vi "Test MQTT-7.1.2-1.vi"(8 "error in (no error)":errorcluster) -> (0 "error out":errorcluster)   [LabVIEW 2013]
uses:
  <vilib>/addons/_JKI Toolkits/Caraya/classes/Test/Test.lvclass
  source/Client/Client.lvclass
  source/MQTT_Base/MQTT_Base.lvclass
  <vilib>/addons/_JKI Toolkits/Caraya/classes/Assert/Assert.lvclass
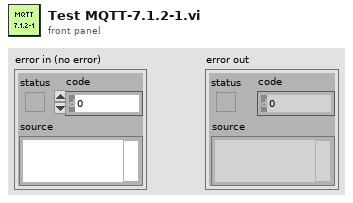
[diagram p1: front panel]
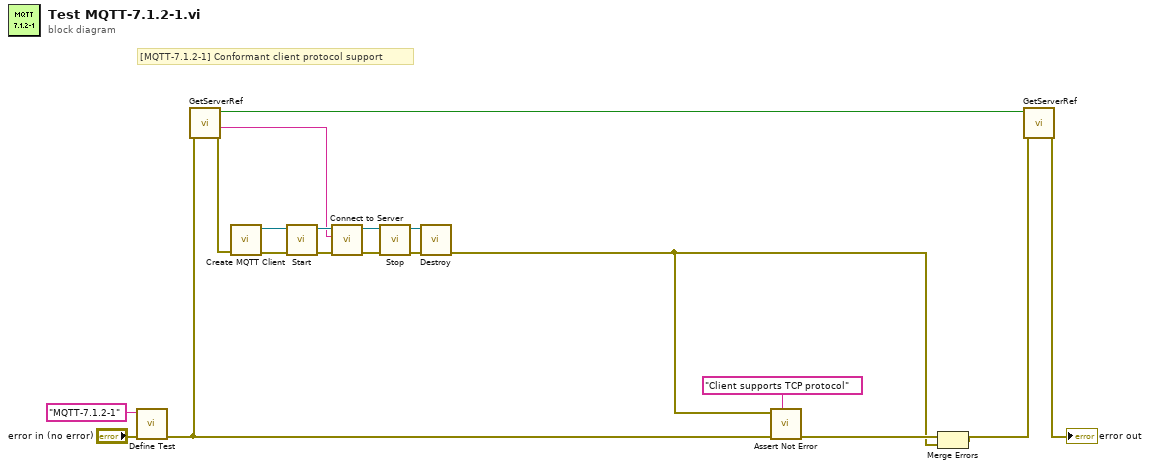
[diagram p0: block diagram]
diagram:
  # "[MQTT-7.1.2-1] Conformant client protocol support"
  n1 = call <vilib>:"Define Test.vi"("error in (no error)"="error in (no error)", "Label (VI Title)"="MQTT-7.1.2-1") -> ("error out"=w5:errorcluster)  [unwired: 9 in]
  n2 = call "GetServerRef.vi"("error in"=w5) -> ("error out"=w16:errorcluster, "Server address"=w4:string, "Created"=w17:bool)  [unwired: 7 in, 1 out]
  n3 = call "Create MQTT Client.vi"("error in (no error)"=w16) -> ("error out"=w8:errorcluster, "Client out"=w9:refnum<class "Client.lvclass">)  [unwired: 9 in]
  n4 = call "Start.vi"("error in (no error)"=w8, "MQTT_Base in"=w9) -> ("error out"=w12:errorcluster, "MQTT_Base out"=w13:refnum<class "Client.lvclass">)  [unwired: 7 in, 1 out]
  n5 = call "Connect to Server.vi"("error in (no error)"=w12, "address (localhost)"=w4, "Client in"=w13) -> ("error out"=w2:errorcluster, "Client out"=w3:refnum<class "Client.lvclass">)  [unwired: 5 in, 2 out]
  n6 = call "Stop.vi"("error in (no error)"=w2, "MQTT_Base in"=w3) -> ("error out"=w10:errorcluster, "MQTT_Base out"=w11:refnum<class "Client.lvclass">)  [unwired: 7 in, 1 out]
  n7 = call "Destroy.vi"("error in (no error)"=w10, "MQTT_Base in"=w11) -> ("error out"=w1:errorcluster)  [unwired: 8 in, 1 out]
  n8 = call <vilib>:"Assert Not Error.vi"("Label"="Client supports TCP protocol", "error in (no error)"=w5, "Not Error?"=w1) -> ("error out"=w6:errorcluster)  [unwired: 8 in]
  n9 = Merge Errors(w6, w1) -> (w7:errorcluster)
  n10 = call "GetServerRef.vi"("error in"=w7, "Destroy (F)"=w17) -> ("error out"=→"error out":errorcluster)  [unwired: 6 in, 3 out]
